vi "Drive_utils_LimitAngle.vi"(3 "Minimum Angle":dbl, 4 "Max Angle Per Iteration":dbl=0.1745, 5 "Angle":dbl, 6 "distance in":dbl) -> (1 "Angle out":dbl, 2 "distance out":dbl)   [LabVIEW 2009, in "Drive.lvlib" / "Drive_Utils.lvlib"]
uses:
  Drive_Utils.lvlib
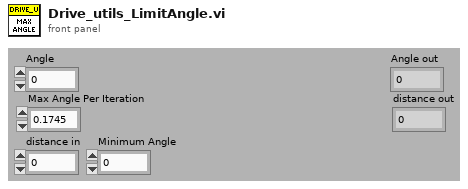
[diagram p1: front panel]
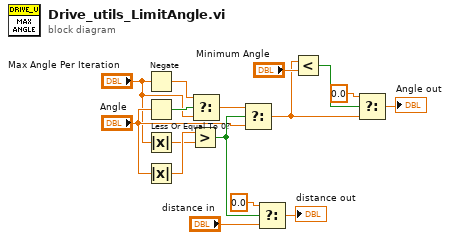
[diagram p0: block diagram]
diagram:
  n1 = Negate(x="Max Angle Per Iteration") -> (-x=w11:dbl)
  n2 = Less Or Equal To 0?(x="Angle") -> (x <= 0?=w12:bool)
  n3 = Absolute Value(x="Max Angle Per Iteration") -> (abs(x)=w6:dbl)
  n4 = Absolute Value(x="Angle") -> (abs(x)=w8:dbl)
  n5 = Greater?(x=w8, y=w6) -> (0:w15:bool)
  n6 = Select(t=w11, s=w12, f="Max Angle Per Iteration") -> (s? t:f=w10:dbl)
  n7 = Select(t=w10, s=w15, f="Angle") -> (s? t:f=w3:dbl)
  n8 = Select(t=0.0, s=w15, f="distance in") -> (s? t:f=→"distance out":dbl)
  n9 = Less?(x=w3, y="Minimum Angle") -> (x < y?=w5:bool)
  n10 = Select(t=0.0, s=w5, f=w3) -> (s? t:f=→"Angle out":dbl)
